vi "Format Key.vi"(10 "Key String":string) -> (2 "Formatted Key":string)   [LabVIEW 2017, in "TOML.lvlib"]
uses:
  TOML.lvlib
  <vilib>/regexp/Match Regular Expression.xnode
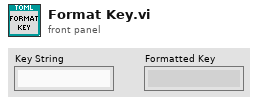
[diagram p1: front panel]
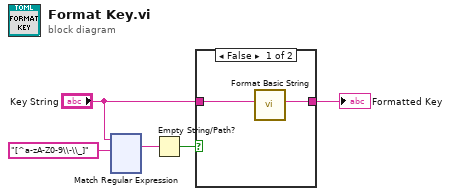
[diagram p0: block diagram]
diagram:
  n1 = xnode "Match Regular Expression"("input string"="Key String", "regular expression"="[^a-zA-Z0-9\\-\\_]") -> ("whole match"=w4:string)  [unwired: 4 in, 4 out]
  n2 = Empty String/Path?(string/path=w4) -> (empty?=w3:bool)
  n3 = case shown="False" w3 {
    tunnel: "Key String" -> [w7 w8]
    tunnel: [w6 w8] -> w1
    frame False {
      n4 = call "Format Basic String.vi"("String"=w7) -> ("Formatted Basic String"=w6:string)  [unwired: 10 in]
    }
    frame True {
    }
  }
  "Formatted Key" <- w1
